vi "Error_Check for Unknow Config Name.vi"(8 "error in (no error)":errorcluster, 11 "Config Name":string) -> (0 "error out":errorcluster)   [LabVIEW 2020]
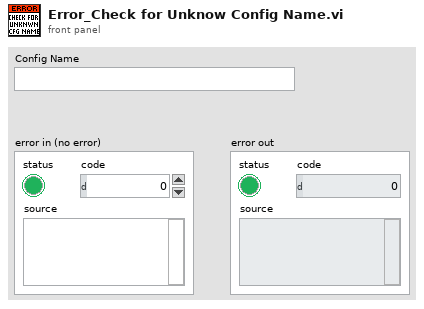
[diagram p1: front panel]
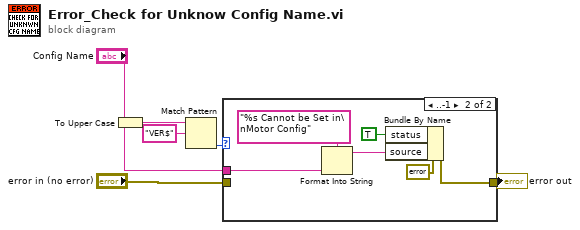
[diagram p0: block diagram]
diagram:
  n1 = To Upper Case(1:"Config Name") -> (0:w1:string)
  n2 = Match Pattern(string=w1, regular expression="VER$") -> (offset past match=w3:i32)  [unwired: 1 in, 3 out]
  n3 = case shown="..-1" w3 {
    tunnel: [w7 w12] -> w5
    tunnel: "Config Name" -> [_ w9]
    tunnel: "error in (no error)" -> [w7 _]
    frame 0.. {
      # "Version"
    }
    frame ..-1 {
      n4 = Format Into String(format string="%s Cannot be Set in\nMotor Config", w9) -> (resulting string=w10:string)  [unwired: 2 in, 1 out]
      n5 = Bundle By Name(cluster=errorcluster {"status"=TRUE, "code"=5000, "source"=""} ("error out"), "status"=TRUE, "source"=w10) -> (w12:errorcluster)
    }
  }
  "error out" <- w5
